vi "instantiate_simple_qa.vi"(0 "vectorestore":refnum<class "abstract_vector_base.lvclass">, 5 "collection_name":string, 7 "chat_model":refnum<class "abstract_llm_base.lvclass">, 9 "embedding_model":refnum<class "abstract_llm_base.lvclass">, 11 "error in (no error)":errorcluster) -> (4 "agent_simple_qa out":refnum<class "agent_simple_qa.lvclass">, 15 "error out":errorcluster)   [LabVIEW 2020, in "agent_simple_qa.lvclass"]
uses:
  agent_simple_qa.lvclass
  models/abstract_llm_base/abstract_llm_base.lvclass
  vectorstore/abstract_vector_base/abstract_vector_base.lvclass
  agent_simple_qa.lvclass/agent_simple_qa.ctl
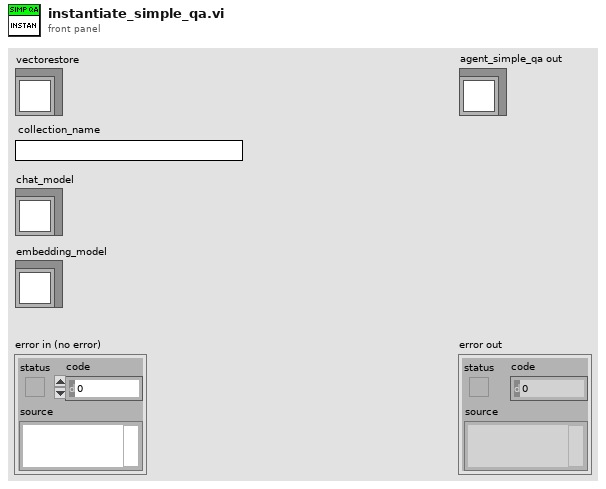
[diagram p1: front panel]
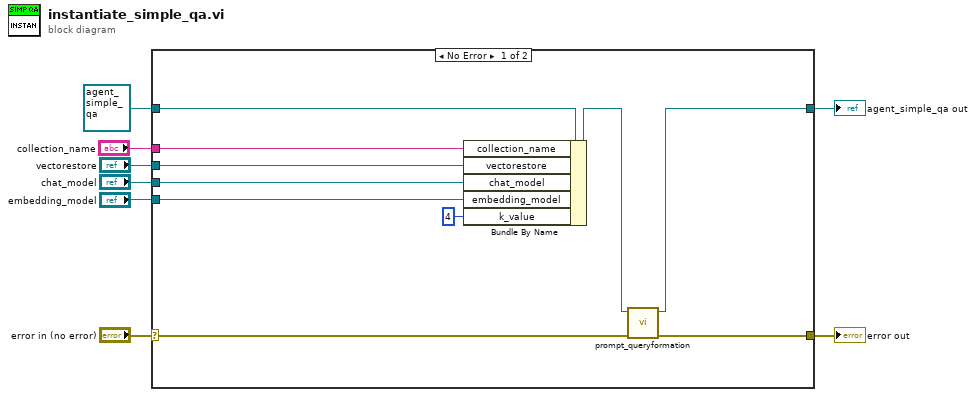
[diagram p0: block diagram]
diagram:
  n1 = case shown="No Error" "error in (no error)" {
    selector: "error in (no error)" -> [w14 w20]
    tunnel: [w12 w20] -> w7
    tunnel: [w11 w19] -> w5
    tunnel: refnum<class "agent_simple_qa.lvclass"> refnum ("agent_simple_qa in") -> [w18 w19]
    tunnel: "vectorestore" -> [w17 _]
    tunnel: "chat_model" -> [w16 _]
    tunnel: "embedding_model" -> [w15 _]
    tunnel: "collection_name" -> [w10 _]
    frame No Error {
      n2 = Bundle By Name(cluster=w18, "collection_name"=w10, "vectorestore"=w17, "chat_model"=w16, "embedding_model"=w15, "k_value"=u32 4) -> (w13:refnum<class "agent_simple_qa.lvclass">)
      n3 = call "prompt_queryformation.vi"("error in (no error)"=w14, "agent_simple_qa in"=w13) -> ("error out"=w12:errorcluster, "agent_simple_qa out"=w11:refnum<class "agent_simple_qa.lvclass">)  [unwired: 8 in]
    }
    frame Error {
    }
  }
  "error out" <- w7
  "agent_simple_qa out" <- w5
